vi "Check logging process is enabled.vi"() -> (3 "Proceed / Logging process is enabled":bool)   [LabVIEW 2020]
uses:
  Typedefs/Set Main VI cursor.ctl
  Global Variables/General Globals.vi
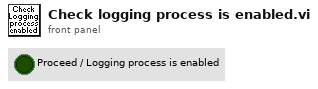
[diagram p1: front panel]
types:
  T1 = typedef "Set Main VI cursor.ctl" = enum16{"Release busy cursor", "Set busy cursor"}
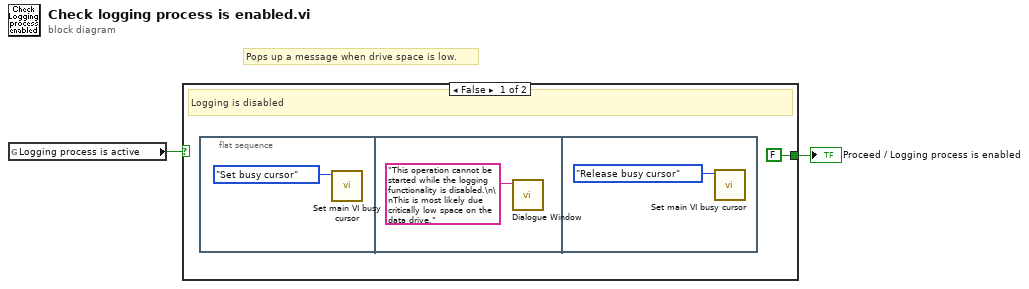
[diagram p0: block diagram]
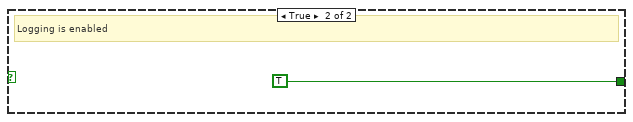
[diagram p2: hidden frame]
diagram:
  # "Pops up a message when drive space is low."
  n1 = global read "General Globals.vi" "Logging process is active"() -> (w1:bool)
  n2 = case shown="False" w1 {
    tunnel: [FALSE TRUE] -> w2
    frame False {
      # "Logging is disabled"
      n3 = flat-sequence {
        frame #0 {
          n4 = call "Set main VI busy cursor.vi"("Main VI's cursor"=Set_Main_VI_cursor."Set busy cursor") -> ()  [unwired: 10 in, 1 out]
        }
        frame #1 {
          n5 = call "Dialogue Window.vi"("Message string"="This operation cannot be started while the logging functionality is disabled.\n\nThis is most likely due critically low space on the data drive.") -> ()  [unwired: 8 in, 3 out]
        }
        frame #2 {
          n6 = call "Set main VI busy cursor.vi"("Main VI's cursor"=Set_Main_VI_cursor."Release busy cursor") -> ()  [unwired: 10 in, 1 out]
        }
      }
    }
    frame True {
      # "Logging is enabled"
    }
  }
  "Proceed / Logging process is enabled" <- w2
